vi "Write configuration.vi"(8 "error in (no error)":errorcluster, 11 "Galvo in":refnum<class "ImagingModeSPIM.lvclass">) -> (0 "error out":errorcluster, 3 "Galvo out":refnum<class "ImagingModeSPIM.lvclass">)   [LabVIEW 2012, in "ImagingModeSPIM.lvclass"]
doc: "Writes the configuration cluster into the configuration file. Configuration file is XML-based. It's name is <component ID>.xml"
uses:
  ImagingModeSPIM.lvclass
  <vilib>/Distrio/Murmex/Murmex/Murmex.lvclass
  ImagingModeSPIM.lvclass/ImagingModeSPIM.ctl
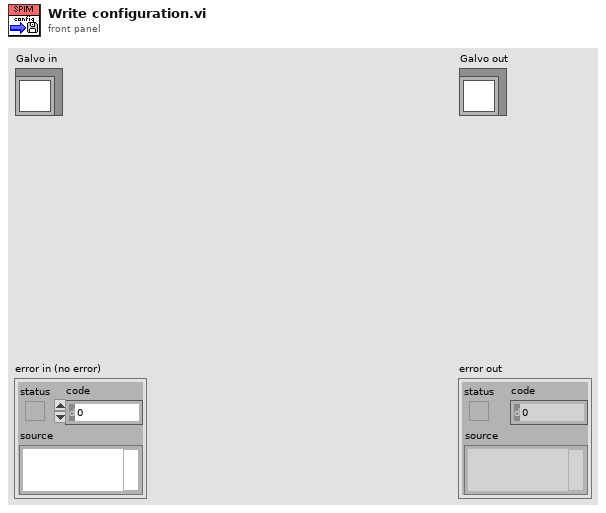
[diagram p1: front panel]
types:
  T1 = typedef "ImagingModeSPIM.lvclass/configuration_cluster.ctl" = cluster{"Sampling rate":dbl, "Samples per channel":i32, "Number of channels":T2, "Task cluster":T3}
  T2 = typedef "ImagingModeSPIM.lvclass/number of channels.ctl" = enum16{"empty", "double sided + PC", "double sided + WFS"}
  T3 = typedef "ImagingModeSPIM.lvclass/task_cluster.ctl" = cluster{"min Voltage":dbl[unit], "max Voltage":dbl[unit], "physical channel":string}
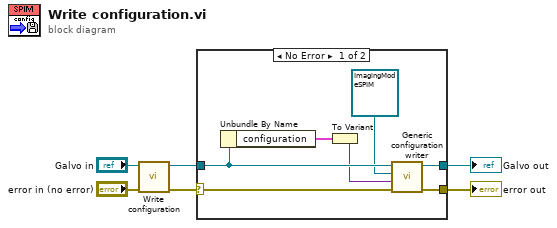
[diagram p0: block diagram]
diagram:
  n1 = call-parent "Write configuration.vi"("error in (no error)"="error in (no error)", "Murmex in"="Galvo in") -> ("error out"=w4:errorcluster, "Murmex out"=w3:refnum<class "ImagingModeSPIM.lvclass">)  [unwired: 8 in]
  n2 = case shown="No Error" w4 {
    selector: w4 -> [w13 w14]
    tunnel: w3 -> [w12 w15]
    tunnel: [w8 w15] -> w2
    tunnel: [w7 w14] -> w1
    frame No Error {
      n3 = Unbundle By Name(w12) -> ("configuration"=w11:T1)
      n4 = To Variant(anything=w11) -> (Variant=w10:variant)
      n5 = call <vilib>:"Generic configuration writer.vi"("error in (no error)"=w13, "configuration"=w10, "inheritance level"=refnum<class "ImagingModeSPIM.lvclass"> refnum ("Galvo.lvclass"), "MurmexBase in"=w12) -> ("error out"=w7:errorcluster, "MurmexBase out"=w8:refnum<class "ImagingModeSPIM.lvclass">)  [unwired: 6 in]
    }
    frame Error {
    }
  }
  "error out" <- w1
  "Galvo out" <- w2
